vi "ErrorCreate.vi"(8 "error in (no error)":errorcluster, 9 "ErrorMessage":string) -> (0 "error out":errorcluster)   [LabVIEW 2016]
doc: "Desoutter controller error handler\n\n(c) 2013 Test & Measurement Solutions. ALL RIGHTS RESERVED\n\nDeveloped by: Test & Measurement Solutions (www.tm-solutions.pl)\nAuthor: Maciej Szupienko (maciej@tm-solutions.pl)\nReleased at: 05th July 2013"
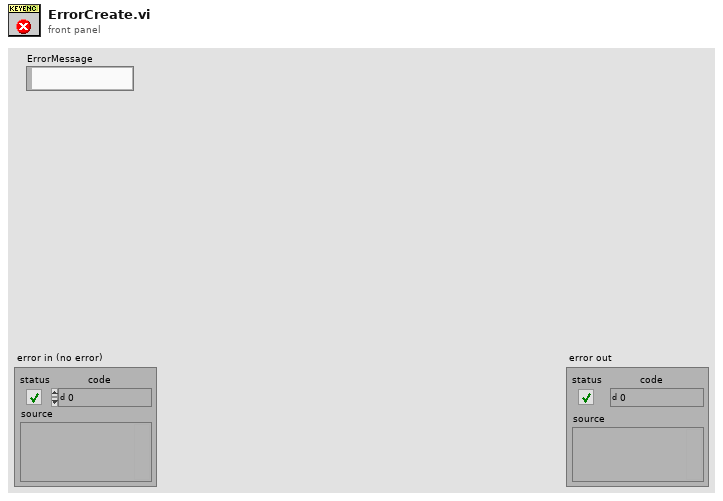
[diagram p1: front panel]
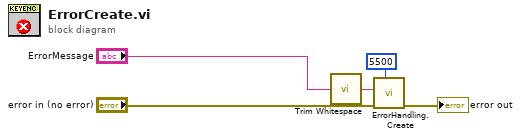
[diagram p0: block diagram]
diagram:
  n1 = call <vilib>:"Trim Whitespace.vi"("string"="ErrorMessage") -> ("trimmed string"=w2:string)  [unwired: 1 in]
  n2 = call "ErrorHandling.Create.vi"("error code (5000)"=5500 ("error code (0)"), "error in"="error in (no error)", "explanation"=w2) -> ("error out"=→"error out":errorcluster)  [unwired: 8 in]
